vi "Set Report Margins.vi"(0 "report in":refnum<class "NI_Word.lvclass">, 5 "margins (1.00)":T1={"top"=1.0, "left"=1.0, "right"=1.0, "bottom"=1.0} {"right" format="%.2f"; "bottom" format="%.2f"; "top" format="%.2f"; "left" format="%.2f"}, 9 "measurement system (default)":u16(ring) items=["Default", "US", "Metric"], 11 "error in (no error)":errorcluster) -> (4 "report out":refnum<class "NI_Word.lvclass">, 10 "page width (Word)":sgl format="%.2f", 15 "error out":errorcluster)   [LabVIEW 2015, in "NI_Word.lvclass"]
doc: "Sets the margins of the specified report."
uses:
  <vilib>/Utility/NIReport.llb/Word/NI_Word.lvclass
  <vilib>/Utility/NIReport.llb/Word/NI_Word.lvclass/NI_Word.ctl
  <vilib>/addons/_office/NI_ReportGenerationToolkit.lvlib
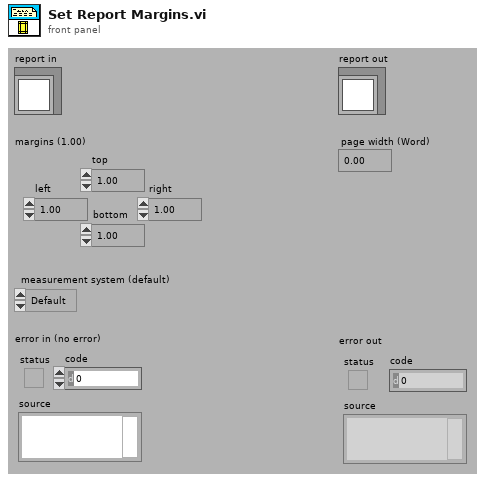
[diagram p1: front panel]
types:
  T1 = cluster{"top":dbl, "left":dbl, "right":dbl, "bottom":dbl}
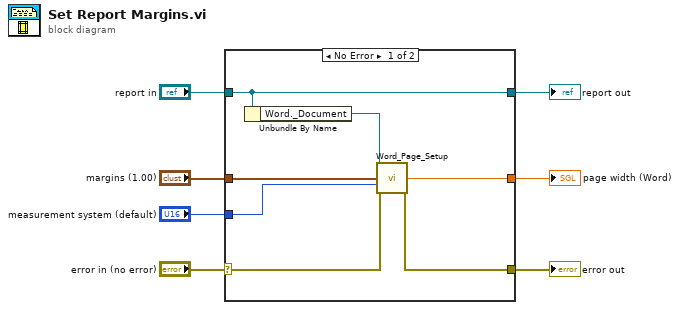
[diagram p0: block diagram]
diagram:
  n1 = case shown="No Error" "error in (no error)" {
    selector: "error in (no error)" -> [w9 w16]
    tunnel: [w8 w16] -> w6
    tunnel: [w13 w15] -> w4
    tunnel: "report in" -> [w13 w15]
    tunnel: "margins (1.00)" -> [w12 _]
    tunnel: "measurement system (default)" -> [w11 _]
    tunnel: [w10 _] -> w1
    frame No Error {
      n2 = Unbundle By Name(w13) -> ("Word._Document"=w14:refnum<k7>)
      n3 = call <vilib>:"Word_Page_Setup.vi"("Word._Document"=w14, "margins (1.00)"=w12, "measurement system (Default)"=w11, "error in"=w9) -> ("page width"=w10:sgl, "error out"=w8:errorcluster)  [unwired: 10 out]
    }
    frame Error {
    }
  }
  "error out" <- w6
  "report out" <- w4
  "page width (Word)" <- w1
